vi "Begin.vi"(11 "Image Size":T4=enum."160x120") -> (0 "error out":errorcluster)   [LabVIEW 2012]
doc: "Called before other user functions, this VI is expected to open initial I/O refnums, load in file data, and do all program initialization. Notice that the <B>error out</B> terminal is simply used for data flow. Wiring it to other structures or subVIs ensures that this VI runs first."
uses:
  <vilib>/Rock Robotics/WPI/Camera/WPI_CameraImageSize.ctl
  <vilib>/Rock Robotics/SystemInterfaces/DIO/FPGA_DIOChannel.ctl
  <vilib>/Rock Robotics/WPI/Encoder/WPI_EncoderType.ctl
  <vilib>/Rock Robotics/SystemInterfaces/Typedef/FPGA_TypedefDigitalModule.ctl
  <vilib>/Rock Robotics/WPI/Camera/WPI_CameraWhite Balance Values.ctl
  <vilib>/Rock Robotics/WPI/Camera/WPI_CameraExposure Values.ctl
  <vilib>/Rock Robotics/WPI/Camera/WPI_CameraFrameRate.ctl
  <vilib>/Rock Robotics/WPI/SafetyOutput/WPI_SafetyOutputConfigMenu.ctl
  <vilib>/Rock Robotics/WPI/DriverStation/WPI_DriverStationRobotMode2.ctl
  <vilib>/Rock Robotics/WPI/Joystick/WPI_JoystickDeviceEnum.ctl
  <vilib>/Rock Robotics/SystemInterfaces/Typedef/FPGA_TypedefAnalogModuleForGyro.ctl
  <vilib>/Rock Robotics/SystemInterfaces/AI/FPGA_AIGyroChannel.ctl
  <vilib>/Rock Robotics/WPI/CAN/Jaguar/SubVIs/WPI_CANJaguar_ControlMode.ctl
  Robot Global Data.vi
  <vilib>/Rock Robotics/WPI/Counter/WPI_CounterDigitalInputToDigitalSource.vi
  <vilib>/Rock Robotics/WPI/Counter/WPI_CounterOpen Gear Tooth Sensor Mode.vi
  <vilib>/Rock Robotics/WPI/MotorControl/WPI_MotorControlOpenCANJaguar.vi
  <vilib>/Rock Robotics/WPI/RobotDrive/WPI_RobotDriveOpen2MotorWithExistingMotors.vi
panel:
  in  "DIO Module":T1
  in  "Invert Direction":bool
  in  "Decoding Type":T2=enum."4x"
  in  "DistancePerCount (deg)":dbl=0.288
  in  "Encoder B Channel":T3=enum."DIO 2"
  in  "Encoder A Channel":T3
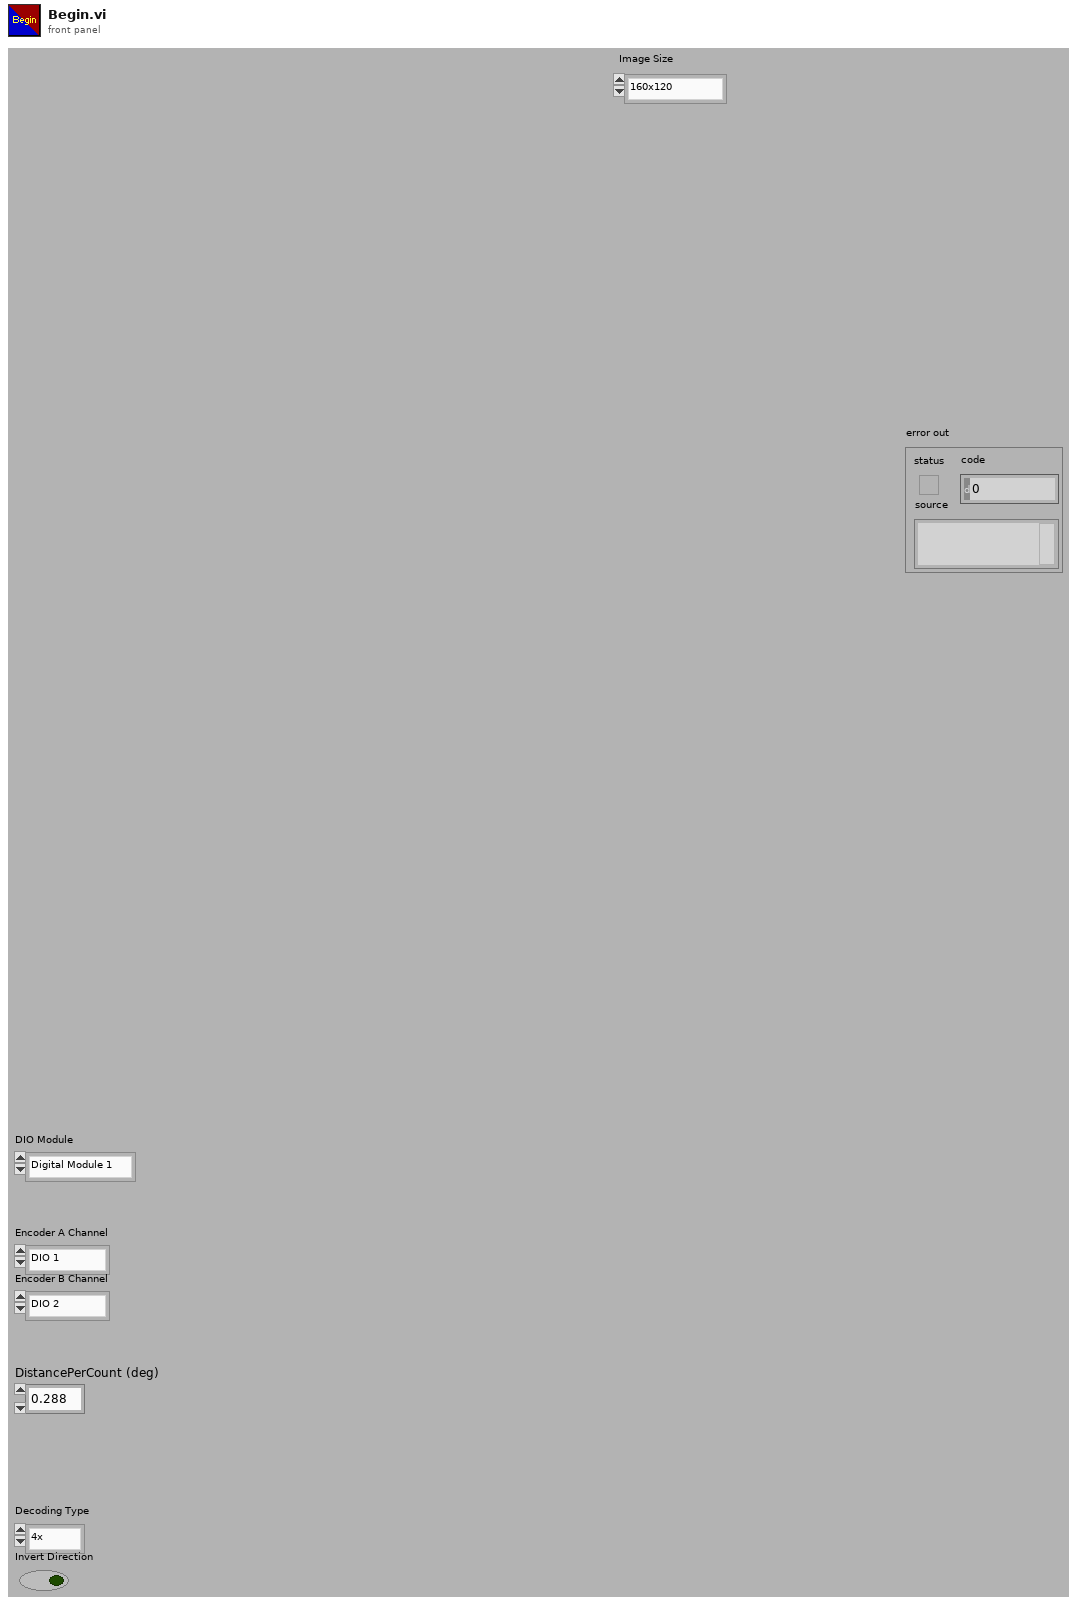
[diagram p1: front panel]
types:
  T1 = typedef "FPGA_TypedefDigitalModule.ctl" = enum16{"Digital Module 1", "Digital Module 2"}
  T2 = typedef "WPI_EncoderType.ctl" = enum16{"1x", "2x", "4x"}
  T3 = typedef "FPGA_DIOChannel.ctl" = enum8{"DIO 1", "DIO 2", "DIO 3", "DIO 4", "DIO 5", "DIO 6", "DIO 7", "DIO 8", "DIO 9", "DIO 10", "DIO 11", "DIO 12", "DIO 13", "DIO 14", "Invalid"}
  T4 = typedef "WPI_CameraImageSize.ctl" = enum16{"640x480", "320x240", "160x120"}
  T5 = typedef "WPI_CANJaguar_ControlMode.ctl" = enum8{"Percent VBus", "Current", "Speed", "Position", "Voltage"}
  T6 = typedef "FPGA_AIGyroChannel.ctl" = enum8{"AI 1", "AI 2", "Invalid"}
  T7 = typedef "FPGA_TypedefAnalogModuleForGyro.ctl" = enum16{"Analog Module 1"}
  T8 = typedef "WPI_JoystickDeviceEnum.ctl" = enum16{"USB 1", "USB 2", "USB 3", "USB 4", "Kinect 1", "Kinect 2"}
  T9 = typedef "WPI_DriverStationRobotMode2.ctl" = enum16{"Autonomous Disabled", "Autonomous Enabled", "Teleop Disabled", "Teleop Enabled", "Timeout", "Finish", "Test Disabled", "Test Enabled"}
  T10 = typedef "WPI_SafetyOutputConfigMenu.ctl" = enum16{"Enable", "Disable"}
  T11 = typedef "WPI_CameraFrameRate.ctl" = u32
  T12 = typedef "WPI_CameraExposure Values.ctl" = enum16{"Auto", "Flicker-free 50 Hz", "Flicker-free 60 Hz", "Hold current"}
  T13 = typedef "WPI_CameraWhite Balance Values.ctl" = enum16{"Auto", "Fixed indoor", "Fixed outdoor 1", "Fixed outdoor 2", "Fixed fluorescent 1", "Fixed fluorescent 2", "Hold current"}
  T14 = typedef "WPI_MotorControlDeviceRef.ctl" = cluster{"DeviceStatus":errorcluster, "Type":enum16{"PWM", "CAN"}, "PWM":cluster{"Digital Module":T1, "PWM Channel":T15, "DeadBand":T16}, "CAN":cluster{"Device Number":u8, "Control Mode":T5, "Semaphore":T17, "Max Vout":dbl}, "Invert":bool, "TransformRef":T18, "InvTransformRef":T18}
  T15 = typedef "FPGA_DIOPWMChannel.ctl" = enum8{"PWM 1", "PWM 2", "PWM 3", "PWM 4", "PWM 5", "PWM 6", "PWM 7", "PWM 8", "PWM 9", "PWM 10", "Invalid"}
  T16 = typedef "WPI_PWMDeadband.ctl" = cluster{"Name":string, "maxPositivePwm":i32, "minPositivePwm":i32, "centerPwm":i32, "maxNegativePwm":i32, "minNegativePwm":i32, "angularRange":u16}
  T17 = typedef "Semaphore RefNum" = refnum<k1>
  T18 = typedef "WPI_PWMTransform_ConPane.ctl" = refnum<vi>
  T19 = typedef "WPI_GyroDevRef.ctl" = cluster{"DevStatus":errorcluster, "Analog Module":T20, "Analog Channel":T21, "Offset":dbl, "Gain (VoltsPerDegree/Second)":dbl}
  T20 = typedef "FPGA_TypedefAnalogModule.ctl" = enum16{"Analog Module 1", "Analog Module 2"}
  T21 = typedef "FPGA_AIChannel.ctl" = enum8{"AI 1", "AI 2", "AI 3", "AI 4", "AI 5", "AI 6", "AI 7", "AI 8", "Invalid"}
  T22 = typedef "WPI_DigitalInputDevRef.ctl" = cluster{"DevStatus":errorcluster, "DIO Channel":T3, "Digital Module":T1}
  T23 = typedef "FPGA_CounterEncoderSourceConvertionLVSourceType.ctl" = cluster{"DevStatus":errorcluster, "AnalogTriggerMode?":bool, "DigitalMode":cluster{"Digital Module":T1, "DIO Channel":T24}, "AnalogTriggerMode":cluster{"AnalogTriggerIndex":T25, "OutputType":T26}}
  T24 = typedef "FPGA_DIODigitalSourceChannel.ctl" = enum8{"DIO 1", "DIO 2", "DIO 3", "DIO 4", "DIO 5", "DIO 6", "DIO 7", "DIO 8", "DIO 9", "DIO 10", "DIO 11", "DIO 12", "DIO 13", "DIO 14", "Disabled"}
  T25 = typedef "FPGA_AnalogTriggerIndex.ctl" = enum8{"Trig 0", "Trig 1", "Trig 2", "Trig 3", "Trig 4", "Trig 5", "Trig 6", "Trig 7", "Invalid"}
  T26 = typedef "FPGA_AnalogTriggerOutType.ctl" = enum16{"InWindow", "TriggerState", "Rising", "Falling"}
  T27 = typedef "WPI_CameraDevRef.ctl" = cluster{"Camera Address":string, "CameraStatus":errorcluster, "Acquire Image Notifier":refnum<notifier>}
  T28 = typedef "WPI_RobotDriveDevRef.ctl" = cluster{"DevStatus":errorcluster, "Motors[]":T14[], "Square Inputs":bool, "Max Output":dbl, "Isochronous":bool}
  T29 = typedef "WPI_JoystickDevRef.ctl" = cluster{"Device":T8}
  T30 = typedef "WPI_EncoderDevRef.ctl" = cluster{"DevStatus":errorcluster, "EncoderIndex":T31, "CounterIndex":T32, "DistancePerCount":dbl, "Decoding Type":T2}
  T31 = typedef "FPGA_EncoderIdx.ctl" = enum8{"Enc 0", "Enc 1", "Enc 2", "Enc 3", "Invalid"}
  T32 = typedef "FPGA_CounterCtrSystemIndex.ctl" = enum8{"Ctr 0", "Ctr 1", "Ctr 2", "Ctr 3", "Ctr 4", "Ctr 5", "Ctr 6", "Ctr 7", "Invalid"}
  T33 = typedef "WPI_CounterDevRef.ctl" = cluster{"DevStatus":errorcluster, "CntIndex":T32}
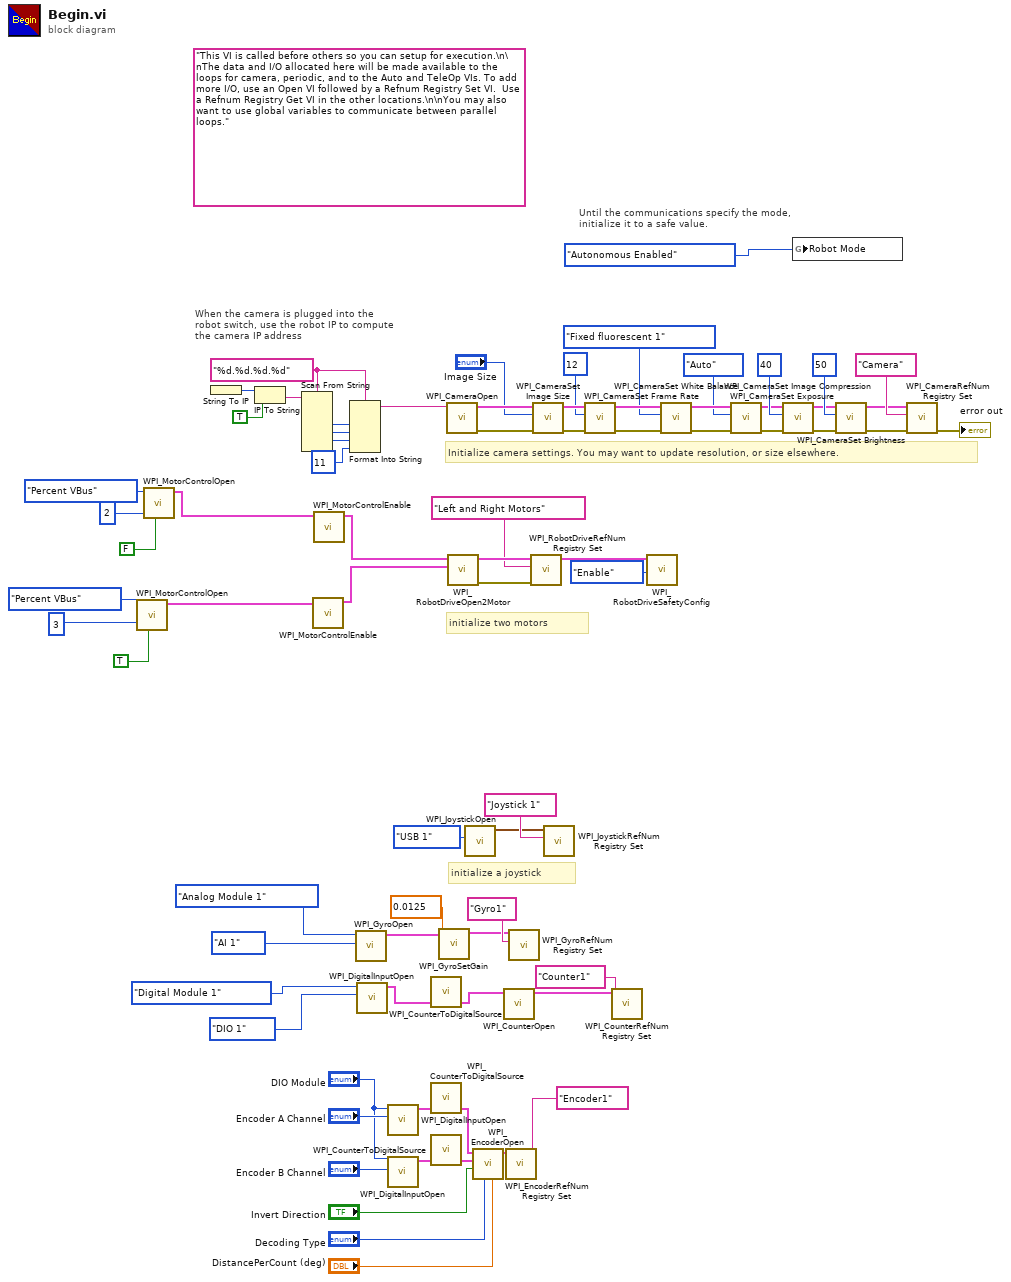
[diagram p0: block diagram]
diagram:
  w43 = "%d.%d.%d.%d" ("format string")
  (unwired) "This VI is called before others so you can setup for execution.\n\nThe data and I/O allocated here will be made available to the loops for camera, periodic, and to the Auto and TeleOp VIs. To add more I/O, use an Open VI followed by a Refnum Registry Set VI.  Use a Refnum Registry Get VI in the other locations.\n\nYou may also want to use global variables to communicate between parallel loops."
  # "initialize a joystick"
  # "Until the communications specify the mode,\ninitialize it to a safe value."
  # "When the camera is plugged into the\nrobot switch, use the robot IP to compute\nthe camera IP address"
  # "initialize two motors"
  # "Initialize camera settings. You may want to update resolution, or size elsewhere."
  n1 = call-poly <vilib>:"WPI_MotorControlOpen.vi"("Invert"=TRUE, "Device Number"=u8 3, "Control Mode"=WPI_CANJaguar_ControlMode."Percent VBus") -> ("MotorControlDeviceRef"=w10:T14)  [unwired: 7 in, 1 out]
  n2 = call-poly <vilib>:"WPI_MotorControlOpen.vi"("Invert"=FALSE, "Device Number"=u8 2, "Control Mode"=WPI_CANJaguar_ControlMode."Percent VBus") -> ("MotorControlDeviceRef"=w9:T14)  [unwired: 7 in, 1 out]
  n3 = String To IP() -> (0:w50:u32)  [unwired: 1 in]
  n4 = IP To String(1:TRUE ("dot notation? (F)"), 2:w50) -> (0:w48:string)
  n5 = Scan From String(format string=w43, input string=w48) -> (output 1=w47:i32, output 2=w46:i32, output 3=w45:i32)  [unwired: 7 in, 3 out]
  n6 = call <vilib>:"WPI_MotorControlEnable.vi"("CAN Jaguar Ref"=w10) -> ("CAN Jaguar Ref Out"=w7:T14)  [unwired: 9 in, 1 out]
  n7 = call <vilib>:"WPI_MotorControlEnable.vi"("CAN Jaguar Ref"=w9) -> ("CAN Jaguar Ref Out"=w8:T14)  [unwired: 9 in, 1 out]
  n8 = Format Into String(format string=w43, w47, w46, w45, 11 ("Compression")) -> (resulting string=w39:string)  [unwired: 2 in, 1 out]
  n9 = call <vilib>:"WPI_GyroOpen.vi"("Analog Channel"=FPGA_AIGyroChannel."AI 1", "Analog Module (Module 1)"=FPGA_TypedefAnalogModuleForGyro."Analog Module 1") -> ("GyroDevRef"=w26:T19)  [unwired: 7 in, 2 out]
  n10 = call <vilib>:"WPI_DigitalInputOpen.vi"("DIO Channel"=FPGA_DIOChannel."DIO 1", "Digital Module (Module 1)"=FPGA_TypedefDigitalModule."Digital Module 1") -> ("DigitalInputDevRef"=w27:T22)  [unwired: 8 in, 1 out]
  n11 = call <vilib>:"WPI_DigitalInputOpen.vi"("DIO Channel"="Encoder A Channel", "Digital Module (Module 1)"="DIO Module") -> ("DigitalInputDevRef"=w20:T22)  [unwired: 1 in, 8 out]
  n12 = call <vilib>:"WPI_DigitalInputOpen.vi"("DIO Channel"="Encoder B Channel", "Digital Module (Module 1)"="DIO Module") -> ("DigitalInputDevRef"=w21:T22)  [unwired: 1 in, 8 out]
  n13 = call-poly <vilib>:"WPI_CounterToDigitalSource.vi"("DigitalInputDevRef"=w27) -> ("Digital Source"=w24:T23)  [unwired: 6 in]
  n14 = call-poly <vilib>:"WPI_CounterToDigitalSource.vi"("DigitalInputDevRef"=w20) -> ("Digital Source"=w19:T23)  [unwired: 6 out]
  n15 = call-poly <vilib>:"WPI_CounterToDigitalSource.vi"("DigitalInputDevRef"=w21) -> ("Digital Source"=w22:T23)  [unwired: 6 out]
  n16 = call <vilib>:"WPI_GyroSetGain.vi"("Gain (VoltsPerDegree/Second)"=0.0125, "GyroDevRef"=w26) -> ("GyroDevRef"=w25:T19)  [unwired: 8 in, 1 out]
  n17 = call <vilib>:"WPI_CameraOpen.vi"("Camera Address"=w39) -> ("error out"=w62:errorcluster, "CameraDevRef"=w63:T27)  [unwired: 1 in, 8 out]
  n18 = call-poly <vilib>:"WPI_RobotDriveOpen2Motor.vi"("Right Motor Dev Ref"=w7, "Left Motor Dev Ref"=w8) -> ("error out"=w71:errorcluster, "RobotDriveDevRef"=w73:T28)  [unwired: 3 in, 5 out]
  n19 = call <vilib>:"WPI_JoystickOpen.vi"("JoystickDevice"=WPI_JoystickDeviceEnum."USB 1") -> ("JoystickDevRef"=w37:T29)  [unwired: 10 in]
  n20 = call <vilib>:"WPI_EncoderOpen.vi"("DistancePerCount"="DistancePerCount (deg)", "Decoding Type"="Decoding Type", "Invert Direction (False)"="Invert Direction", "BSource"=w22, "ASource"=w19) -> ("EncoderDevRef"=w13:T30)  [unwired: 3 in, 3 out]
  n21 = call-poly <vilib>:"WPI_CounterOpen.vi"("Source"=w24) -> ("CounterDevRef"=w23:T33)  [unwired: 9 in, 1 out]
  n22 = call <vilib>:"WPI_EncoderRefNum Registry Set.vi"("refnum name"="Encoder1", "EncoderDevRef"=w13) -> ()  [unwired: 8 in, 2 out]
  n23 = call <vilib>:"WPI_GyroRefNum Registry Set.vi"("refnum name"="Gyro1", "GyroDevRef"=w25) -> ()  [unwired: 8 in, 2 out]
  n24 = call <vilib>:"WPI_RobotDriveRefNum Registry Set.vi"("error in (no error)"=w71, "refnum name"="Left and Right Motors", "RobotDriveDevRef"=w73) -> ("RobotDriveDevRef"=w42:T28)  [unwired: 8 out]
  n25 = call <vilib>:"WPI_CameraSet Image Size.vi"("error in (no error)"=w62, "Image Size"="Image Size", "CameraDevRef"=w63) -> ("error out"=w61:errorcluster, "CameraDevRef Out"=w64:T27)  [unwired: 7 out]
  n26 = call <vilib>:"WPI_JoystickRefNum Registry Set.vi"("refnum name"="Joystick 1", "JoystickDevRef"=w37) -> ()  [unwired: 8 in, 2 out]
  n27 = call <vilib>:"WPI_CameraSet Frame Rate.vi"("error in (no error)"=w61, "Frame Rate (fps)"=T11 12, "CameraDevRef"=w64) -> ("error out"=w60:errorcluster, "CameraDevRef Out"=w66:T27)  [unwired: 7 out]
  n28 = call <vilib>:"WPI_CounterRefNum Registry Set.vi"("refnum name"="Counter1", "CounterDevRef"=w23) -> ()  [unwired: 8 in, 2 out]
  n29 = call <vilib>:"WPI_RobotDriveSafetyConfig.vi"("mode"=WPI_SafetyOutputConfigMenu."Enable", "RobotDriveDevRef"=w42) -> ()  [unwired: 8 in, 2 out]
  n30 = call <vilib>:"WPI_CameraSet White Balance.vi"("error in (no error)"=w60, "White Balance"=WPI_CameraWhite_Balance_Values."Fixed fluorescent 1", "CameraDevRef"=w66) -> ("error out"=w59:errorcluster, "CameraDevRef Out"=w65:T27)  [unwired: 7 out]
  n31 = call <vilib>:"WPI_CameraSet Exposure.vi"("error in (no error)"=w59, "Exposure"=WPI_CameraExposure_Values."Auto", "CameraDevRef"=w65) -> ("error out"=w58:errorcluster, "CameraDevRef Out"=w68:T27)  [unwired: 7 out]
  n32 = call <vilib>:"WPI_CameraSet Image Compression.vi"("error in (no error)"=w58, "Compression"=40, "CameraDevRef"=w68) -> ("error out"=w57:errorcluster, "CameraDevRef Out"=w67:T27)  [unwired: 7 out]
  n33 = global write "Robot Global Data.vi" "Robot Mode"(WPI_DriverStationRobotMode2."Autonomous Enabled" ("Robot Mode")) -> ()
  n34 = call <vilib>:"WPI_CameraSet Brightness.vi"("error in (no error)"=w57, "Brightness"=50, "CameraDevRef"=w67) -> ("error out"=w55:errorcluster, "CameraDevRef Out"=w56:T27)  [unwired: 7 out]
  n35 = call <vilib>:"WPI_CameraRefNum Registry Set.vi"("error in (no error)"=w55, "refnum name"="Camera", "CameraDevRef"=w56) -> ("error out"=→"error out":errorcluster)  [unwired: 8 out]
